vi "Coerce and Warning.vi"(0 "Max":dbl, 1 "Name":string, 5 "Value in":dbl, 7 "Min":dbl, 9 "coerce?":bool=TRUE, 11 "error in":errorcluster) -> (6 "Value out":dbl, 15 "error out":errorcluster)   [LabVIEW 2015]
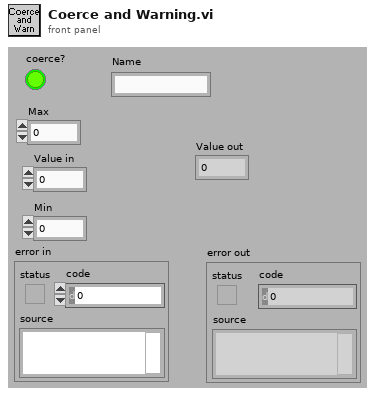
[diagram p1: front panel]
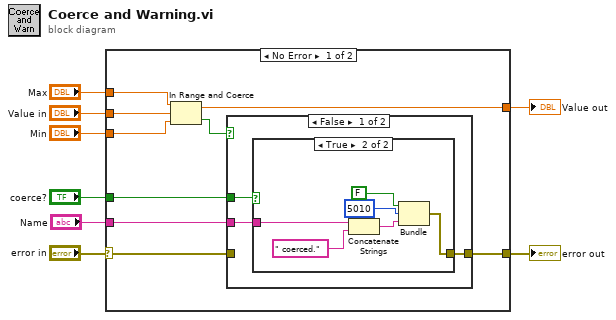
[diagram p0: block diagram]
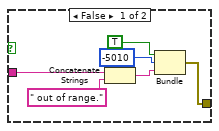
[diagram p2: hidden frame]
diagram:
  n1 = case shown="No Error" "error in" {
    selector: "error in" -> [w12 w35]
    tunnel: [w11 w35] -> w7
    tunnel: "Max" -> [w17 _]
    tunnel: "Value in" -> [w15 w34]
    tunnel: "Min" -> [w16 _]
    tunnel: "coerce?" -> [w10 _]
    tunnel: "Name" -> [w9 _]
    tunnel: [w14 w34] -> w1
    frame No Error {
      n2 = In Range and Coerce(upper limit=w17, x=w15, lower limit=w16) -> (coerced(x)=w14:dbl, In Range?=w13:bool)
      n3 = case shown="False" w13 {
        tunnel: [w18 w33] -> w11
        tunnel: w12 -> [_ w33]
        tunnel: w10 -> [w20 _]
        tunnel: w9 -> [w19 _]
        frame False {
          n4 = case shown="True" w20 {
            tunnel: w19 -> [w26 w28]
            tunnel: [w21 w27] -> w18
            frame False {
              n5 = Concatenate Strings(w26, " out of range.") -> (w22:string)
              n6 = Bundle(TRUE, -5010, w22) -> (w21:errorcluster)  [unwired: 1 in]
            }
            frame True {
              n7 = Concatenate Strings(w28, " coerced.") -> (w29:string)
              n8 = Bundle(FALSE, 5010, w29) -> (w27:errorcluster)  [unwired: 1 in]
            }
          }
        }
        frame True {
        }
      }
    }
    frame Error {
    }
  }
  "error out" <- w7
  "Value out" <- w1
